vi "Result_Test.vi"(8 "error in (no error)":errorcluster caption="entrée d'erreur (pas d'erreur)", 11 "Flash_Jlink en entrée":refnum<class "P2265_SwitchOn_Test.lvclass">) -> (0 "error out":errorcluster caption="sortie d'erreur", 3 "Flash_Jlink en sortie":refnum<class "P2265_SwitchOn_Test.lvclass">)   [LabVIEW 2020, in "Library Test.lvlib" / "P2265_SwitchOn_Test.lvclass"]
uses:
  P2265_SwitchOn_Test.lvclass
  C:/Users/ngarcin/OneDrive - Altyor/Standard TB/Class/Test/Test (Default)/Test (Default).lvclass
  JSON API/JSON Value/Set from JSON string.vi
  JSON API/JSON Value/JSON Value.lvclass
  Test_Wtih_Instr/Test_With_Inst.lvclass
  P2265_SwitchOn_Test.lvclass/P2265_SwitchOn_Test.ctl
  JSON API/Variant JSON/Variant JSON.lvlib
  JSON API/Get Polymorphic/JSON GetSet.lvlib
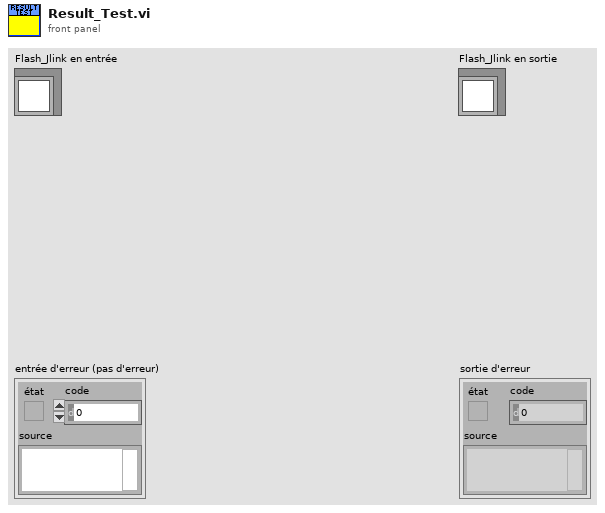
[diagram p1: front panel]
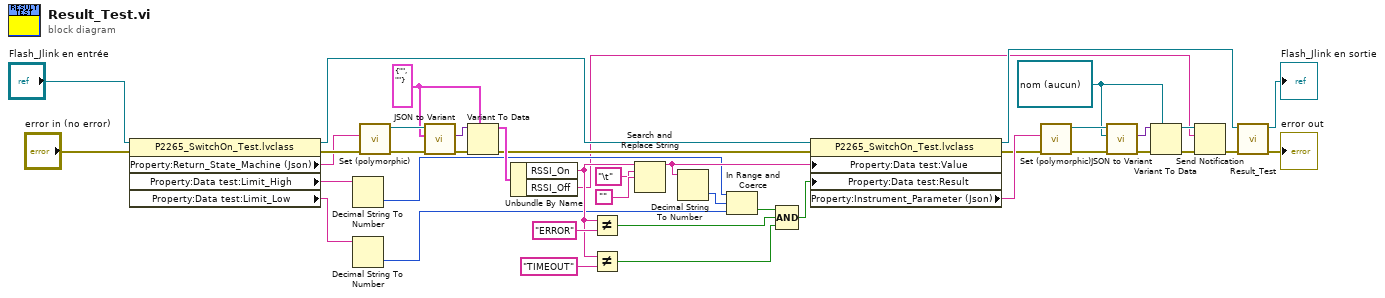
[diagram p0: block diagram]
diagram:
  w19 = cluster{"RSSI_On":string, "RSSI_Off":string} {"RSSI_On"="", "RSSI_Off"=""} ("Cluster des données privées de classe")
  w27 = refnum<notifier> refnum ("notificateur en sortie")
  n1 = property class="P2265_SwitchOn_Test.lvclass"(reference="Flash_Jlink en entrée", error in="error in (no error)") -> (reference out=w15:refnum<class "P2265_SwitchOn_Test.lvclass">, error out=w14:errorcluster, "Property:Return_State_Machine (Json)"=w12:string, "Property:Data test:Limit_High"=w7:string, "Property:Data test:Limit_Low"=w6:string)
  n2 = Decimal String To Number(string=w7) -> (number=w4:i32)  [unwired: 2 in, 1 out]
  n3 = Decimal String To Number(string=w6) -> (number=w5:i32)  [unwired: 2 in, 1 out]
  n4 = call-poly "Set (polymorphic).vi"("error in (no error)"=w14, "JSON stream"=w12) -> ("error out"=w21:errorcluster, "JSON Value out"=w23:refnum<class "JSON Value.lvclass">)  [unwired: 7 in, 1 out]
  n5 = call "JSON to Variant.vi"("error in (no error)"=w21, "Variant (Data Type)"=w19, "JSON Value"=w23) -> ("error out"=w22:errorcluster, "Variant out"=w20:variant)  [unwired: 7 in]
  n6 = Variant To Data(error in=w22, type=w19, Variant=w20) -> (data=w18:cluster{"RSSI_On":string, "RSSI_Off":string}, error out=w17:errorcluster)
  n7 = Unbundle By Name(w18) -> ("RSSI_On"=w9:string, "RSSI_Off"=w1:string)
  n8 = Not Equal?(x=w9, y="ERROR" ("expression régulière")) -> (x != y?=w36:bool)
  n9 = Not Equal?(x=w9, y="TIMEOUT" ("expression régulière")) -> (x != y?=w35:bool)
  n10 = Search and Replace String(input string=w9, search string="\t", replace string="") -> (result string=w8:string)  [unwired: 5 in, 3 out]
  n11 = Decimal String To Number(string=w8) -> (number=w3:i32)  [unwired: 2 in, 1 out]
  n12 = In Range and Coerce(upper limit=w4, x=w3, lower limit=w5) -> (In Range?=w2:bool)  [unwired: 1 out]
  n13 = Compound Arithmetic op=AND ("Opérateur arithmétique")(w2, w36, w35) -> (w34:bool)
  n14 = property class="P2265_SwitchOn_Test.lvclass"(reference=w15, error in=w17, "Property:Data test:Value"=w8, "Property:Data test:Result"=w34) -> (reference out=w39:refnum<class "P2265_SwitchOn_Test.lvclass">, error out=w28:errorcluster, "Property:Instrument_Parameter (Json)"=w29:string)
  n15 = call-poly "Set (polymorphic).vi"("error in (no error)"=w28, "JSON stream"=w29) -> ("error out"=w31:errorcluster, "JSON Value out"=w33:refnum<class "JSON Value.lvclass">)  [unwired: 7 in, 1 out]
  n16 = call "JSON to Variant.vi"("error in (no error)"=w31, "Variant (Data Type)"=w27, "JSON Value"=w33) -> ("error out"=w32:errorcluster, "Variant out"=w30:variant)  [unwired: 7 in]
  n17 = Variant To Data(error in=w32, type=w27, Variant=w30) -> (data=w24:refnum<notifier>, error out=w26:errorcluster)
  n18 = Send Notification(notification=w1, notifier=w24, error in (no error)=w26) -> (error out=w25:errorcluster)  [unwired: 1 out]
  n19 = call-parent "Result_Test.vi"("error in (no error)"=w25, "Test_With_Inst en entrée"=w39) -> ("error out"=→"error out":errorcluster, "Test_With_Inst en sortie"=→"Flash_Jlink en sortie":refnum<class "P2265_SwitchOn_Test.lvclass">)  [unwired: 8 in]
